vi "Periodic Tasks.vi"(8 "error in":errorcluster) -> ()   [LabVIEW 2018]
doc: "This VI runs in parallel to other robot code. It can contain as many user-defined periodic loops as you need. These can carry out PID or other sorts of timed response."
uses:
  <vilib>/Rock Robotics/WPI/Utilities/WPI_GetSetVariantRefNum.vi
  Robot Global Data.vi
panel:
  out "all currents (A) 2":dbl[](array[numeric]) caption="0\n1\n2\n3\n4\n5\n6\n7\n8\n9\n10\n11\n12\n13\n14\n15"
  out "Solenoid Voltage":dbl
  out "Input Voltage":dbl
  out "Compressor current (A)":dbl
  out "all currents (A)":dbl[](array[numeric]) caption="0\n1\n2\n3\n4\n5\n6\n7\n8\n9\n10\n11\n12\n13\n14\n15"
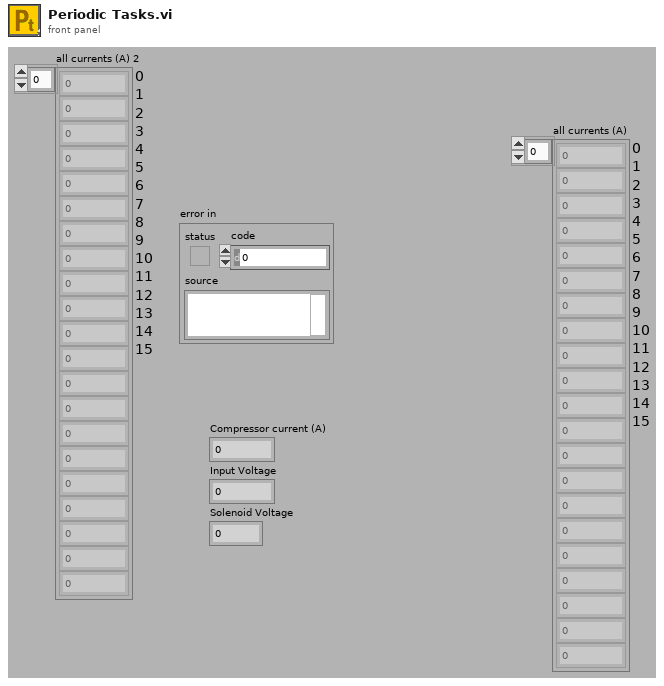
[diagram p1: front panel]
types:
  T1 = typedef "Command Status Info.ctl" = cluster{"Name":string, "Status":T2, "notifier out":T3}
  T2 = typedef "Completion Status.ctl" = enum16{"Successful", "Aborted", "Incomplete"}
  T3 = typedef "Completion Notifier.ctl" = refnum<notifier>
  T4 = typedef "WPI_JoystickDevRef.ctl" = cluster{"Device":T5}
  T5 = typedef "WPI_JoystickDeviceEnum.ctl" = enum16{"USB 0", "USB 1", "USB 2", "USB 3", "USB 4", "USB 5"}
  T6 = cluster{"JoystickDevRef":T4, "JoystickDevRef":T4}
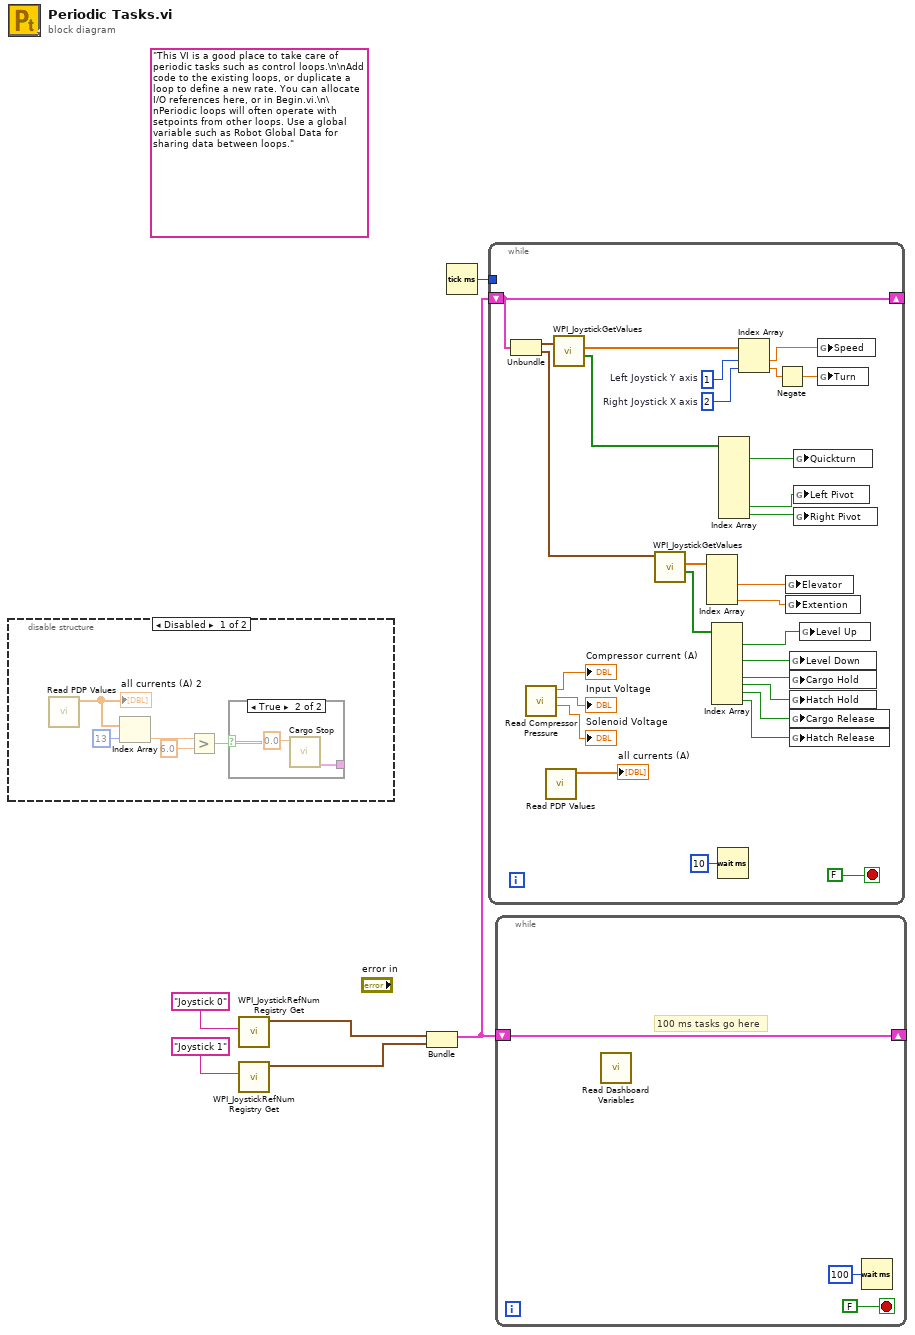
[diagram p0: block diagram]
diagram:
  (unwired) "This VI is a good place to take care of periodic tasks such as control loops.\n\nAdd code to the existing loops, or duplicate a loop to define a new rate. You can allocate I/O references here, or in Begin.vi.\n\nPeriodic loops will often operate with setpoints from other loops. Use a global variable such as Robot Global Data for sharing data between loops."
  n1 = disable-structure shown="Disabled" {
    frame Disabled {
      n2 = call "Read PDP Values.vi"() -> ("all currents (A)"=w8:dbl[])  [unwired: 11 in]
      "all currents (A) 2" <- w8
      n3 = Index Array(array=w8, index=13) -> (element=w10:dbl)
      n4 = Greater?(x=w10, y=6.0) -> (0:w7:bool)
      n5 = case shown="True" w7 {
        tunnel: [_ w13] -> _
        frame False {
        }
        frame True {
          n6 = call "Cargo Stop.vi"("Setpoint"=0.0) -> ("Command Info Out"=w13:T1)  [unwired: 10 in]
        }
      }
    }
    frame Enabled {
    }
  }
  n7 = call <vilib>:"WPI_JoystickRefNum Registry Get.vi"("refnum name"="Joystick 0") -> ("JoystickDevRef"=w3:T4)  [unwired: 1 in, 9 out]
  n8 = call <vilib>:"WPI_JoystickRefNum Registry Get.vi"("refnum name"="Joystick 1") -> ("JoystickDevRef"=w1:T4)  [unwired: 1 in, 9 out]
  n9 = Bundle("JoystickDevRef"=w3, "JoystickDevRef"=w1) -> (w2:T6)  [unwired: 1 in]
  n10 = Tick Count (ms)() -> (millisecond timer value=w5:u32)
  n11 = while {
    shift-right: [w34] -> _
    shift-left: w2 -> [w34]
    tunnel: w5 -> [_]
    stop <- FALSE stop-if-true
    w20 = 2  # Right Joystick X axis
    w21 = 1  # Left Joystick Y axis
    n12 = Unbundle(w34) -> ("JoystickDevRef"=w33:T4, "JoystickDevRef"=w30:T4)
    n13 = call "Read Compressor Pressure.vi"() -> ("Solenoid Voltage"=→"Solenoid Voltage":dbl, "Input Voltage"=→"Input Voltage":dbl, "Compressor current (A)"=→"Compressor current (A)":dbl)  [unwired: 9 in]
    n14 = call "Read PDP Values.vi"() -> ("all currents (A)"=→"all currents (A)":dbl[])  [unwired: 11 in]
    n15 = call <vilib>:"WPI_JoystickGetValues.vi"("JoystickDevRef"=w33) -> ("Buttons"=w38:bool[], "Axes"=w40:dbl[])  [unwired: 6 in, 3 out]
    n16 = call <vilib>:"WPI_JoystickGetValues.vi"("JoystickDevRef"=w30) -> ("Buttons"=w32:bool[], "Axes"=w31:dbl[])  [unwired: 6 in, 3 out]
    n17 = Index Array(array=w31) -> (element #2=w23:dbl, element #4=w22:dbl)  [unwired: 4 in, 2 out]
    n18 = Index Array(array=w32) -> (element #1=w28:bool, element #3=w27:bool, element #5=w24:bool, element #6=w29:bool, element #7=w26:bool, element #8=w25:bool)  [unwired: 8 in, 2 out]
    n19 = Wait (ms)(milliseconds to wait=u32 10) -> ()  [unwired: 1 out]
    n20 = Index Array(array=w38) -> (element #1=w37:bool, element #7=w36:bool, element #8=w35:bool)  [unwired: 8 in, 5 out]
    n21 = Index Array(array=w40, index #1=w21, index #2=w20) -> (element #1=w19:dbl, element #2=w18:dbl)
    n22 = Negate(x=w18) -> (-x=w39:dbl)
    n23 = global write "Robot Global Data.vi" "Elevator"(w23) -> ()
    n24 = global write "Robot Global Data.vi" "Extention"(w22) -> ()
    n25 = global write "Robot Global Data.vi" "Level Down"(w27) -> ()
    n26 = global write "Robot Global Data.vi" "Cargo Hold"(w24) -> ()
    n27 = global write "Robot Global Data.vi" "Hatch Hold"(w29) -> ()
    n28 = global write "Robot Global Data.vi" "Cargo Release"(w26) -> ()
    n29 = global write "Robot Global Data.vi" "Hatch Release"(w25) -> ()
    n30 = global write "Robot Global Data.vi" "Quickturn"(w37) -> ()
    n31 = global write "Robot Global Data.vi" "Left Pivot"(w36) -> ()
    n32 = global write "Robot Global Data.vi" "Right Pivot"(w35) -> ()
    n33 = global write "Robot Global Data.vi" "Level Up"(w28) -> ()
    n34 = global write "Robot Global Data.vi" "Speed"(w19) -> ()
    n35 = global write "Robot Global Data.vi" "Turn"(w39) -> ()
  }
  n36 = while {
    shift-right: [w43] -> _
    shift-left: w2 -> [w43]
    stop <- FALSE stop-if-true
    # "100 ms tasks go here"
    n37 = call "Read Dashboard Variables.vi"() -> ()  [unwired: 12 in]
    n38 = Wait (ms)(milliseconds to wait=u32 100) -> ()  [unwired: 1 out]
  }
